vi "Disconnect.vi"(8 "error in":errorcluster, 11 "IF_XX in":refnum<class "IF_XX.lvclass">) -> (0 "error out":errorcluster, 3 "IF_XX out":refnum<class "IF_XX.lvclass">)   [LabVIEW 2019, in "IF_XX.lvlib" / "IF_XX.lvclass"]
doc: "This disconnect routine is a must override from the Instrument Class\nChildren Classes are responsible for handling the override, but the parent class is an intermediary and must contain the override functions to maintain the rules for the method."
uses:
  Library/IF_XX.lvclass
  Library/IF_XX.lvclass/IF_XX.ctl
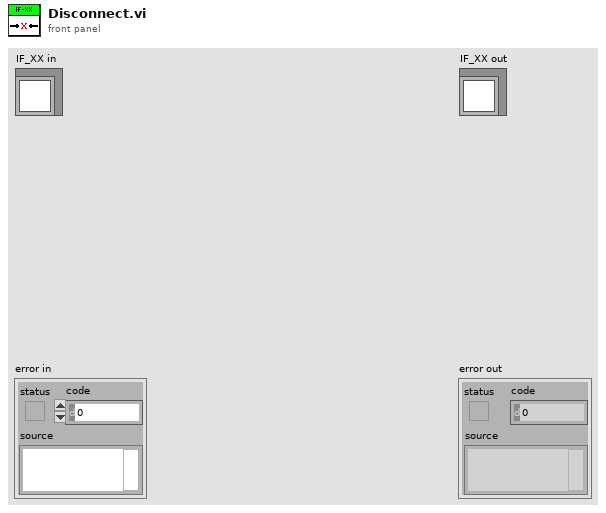
[diagram p1: front panel]
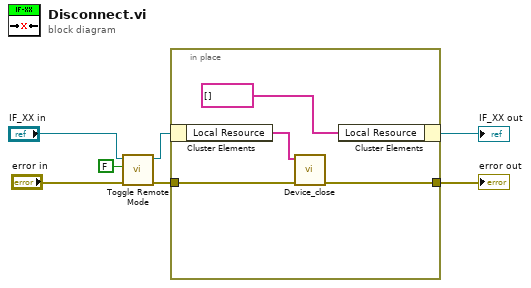
[diagram p0: block diagram]
diagram:
  n1 = call "Toggle Remote Mode.vi"("error in (no error)"="error in", "Remote"=FALSE, "IF_XX in"="IF_XX in") -> ("error out"=w3:errorcluster, "IF_XX out"=w2:refnum<class "IF_XX.lvclass">)  [unwired: 7 in]
  n2 = in-place {
    in-place-border: w3 -> [w10]
    in-place-border: [w9] -> w6
    n3 = in-place-cluster #1(w2) -> ("Local Resource"=w11:string[])
    n4 = call <instrlib>:"Device_close.vi"("error in (no error)"=w10, "Device information in"=w11) -> ("Fehler (Ausgang)"=w9:errorcluster)  [unwired: 3 in]
    n5 = in-place-cluster #1("Local Resource"=string[] []) -> (→"IF_XX out":refnum<class "IF_XX.lvclass">)
  }
  "error out" <- w6
